vi "Save_EEG_To_XML.vi"(0 "Path to EEG File":path, 1 "SampleRateHz":dbl, 2 "Epoch Duration":dbl, 5 "EEG Refnum in":refnum<data-value>, 7 "ChannelNames in":string[](array[string]), 9 "Trial Info":T1, 11 "error in (no error)":errorcluster) -> (6 "EEG Refnum out":refnum<data-value>, 15 "error out":errorcluster)   [LabVIEW 2016, in "Save Txt To Xml.lvlib"]
uses:
  Save Txt To Xml.lvlib
  Trial_Info.ctl
  _XML_EEG_File_Parser/_vlib/XML_EEG_File.lvclass
  _XML_EEG_File_Parser/_vlib/XML_EEG_Header.ctl
  _XML_EEG_File_Parser/_vlib/XML_EEG_Dataset.ctl
  <vilib>/Waveform/WDTOps.llb/WDT Get Waveform Subset DBL.vi
  <vilib>/measure/madcrms.llb/Basic Averaged DC-RMS for 1 Chan.vi
  _XML_EEG_File_Parser/XML_EEG_File_Parser.lvlib
  <vilib>/measure/NI_MAPro.lvlib
panel:
  # "This VI is a part of BCI Design library, http://www.ru-bci.org \nCopyright © 2020, Sotnikov Peter, All rights reserved. License: GNU GPLv3"
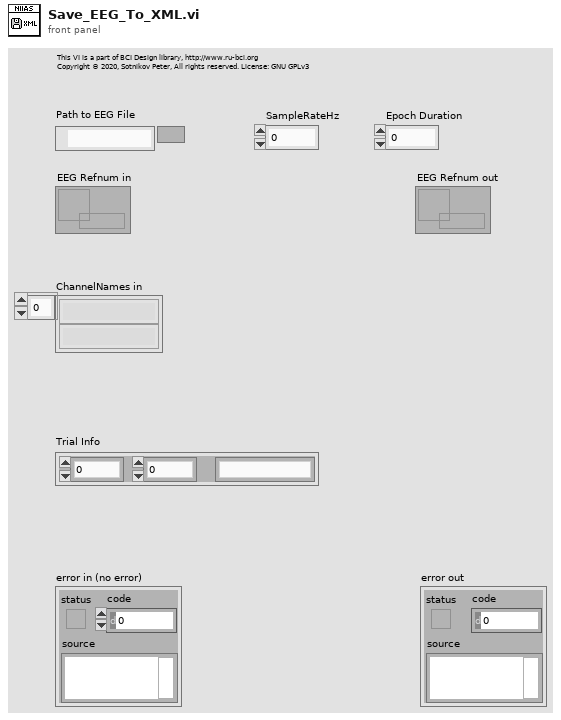
[diagram p1: front panel]
types:
  T1 = typedef "Save Txt To Xml.lvlib/Trial_Info.ctl" = cluster{"Start Position":i32, "End Position":i32, "Class":string}
  T2 = typedef "XML_EEG_File_Parser.lvlib/XML_EEG_Dataset.ctl" = cluster{"Attributes":cluster{"NumberOfSamples":i32, "StartDateTime":timestamp}, "Body":cluster{"MarkerValue":string, "Channels":waveform(dbl)[]}}
  T3 = typedef "XML_EEG_File_Parser.lvlib/XML_EEG_Header.ctl" = cluster{"Attributes":cluster{"ChannelDataType":string, "NumberOfChannels":i32, "SampleRateHz":dbl, "MarkerChannel":i32}, "Body":cluster{"PatientSpecificData":string, "NumberOfDatasets":i32, "Channels":string[]}}
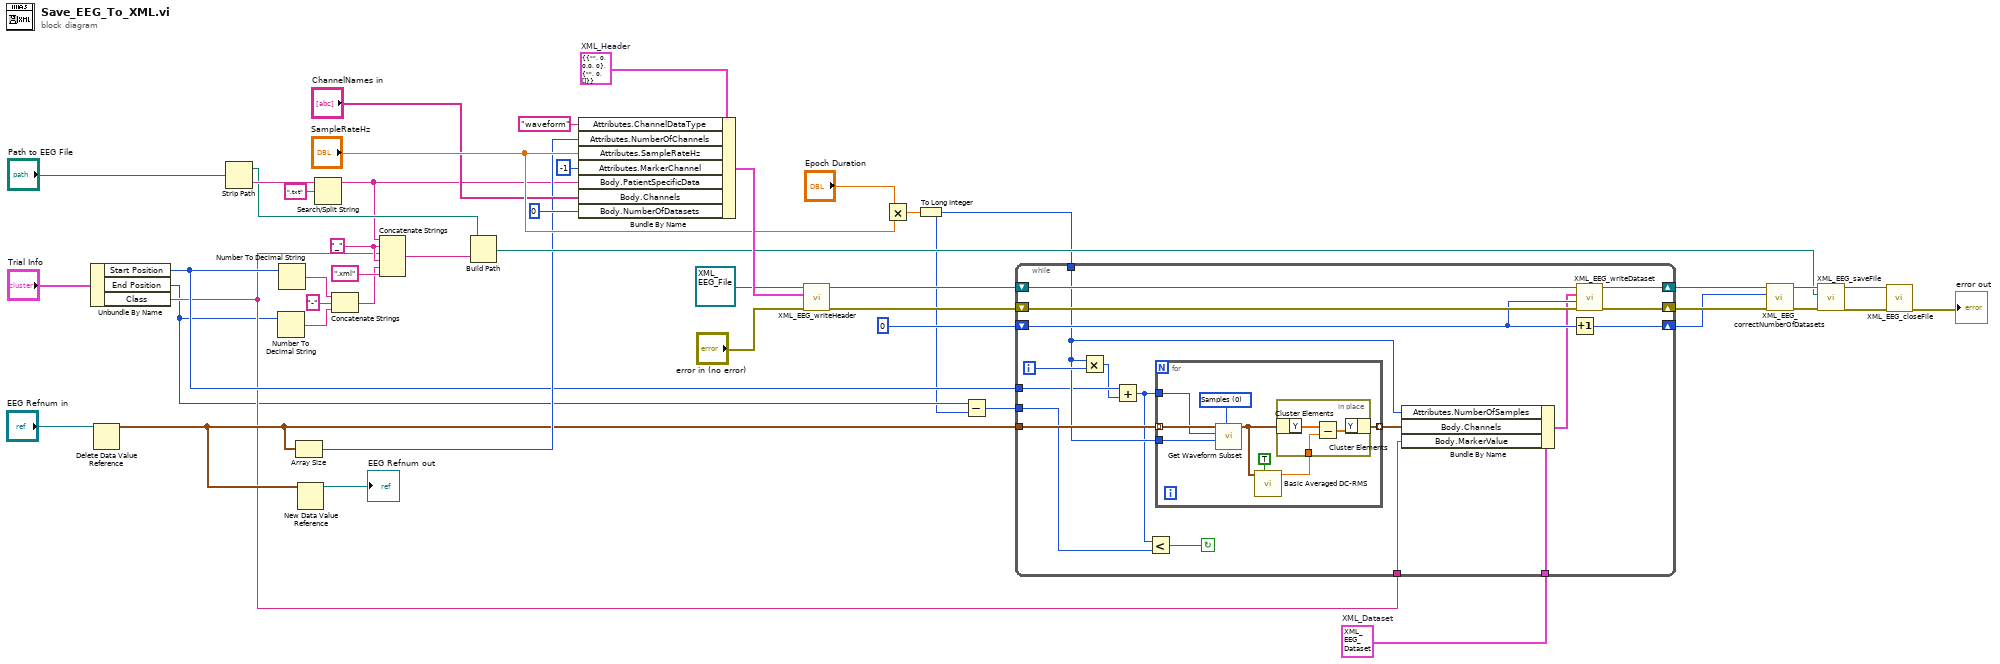
[diagram p0: block diagram]
diagram:
  w9 = "_" ("string")
  w34 = T2 {"Attributes"={"NumberOfSamples"=0, "StartDateTime"=timestamp(0 s since 1904-01-01)}, "Body"={"MarkerValue"="", "Channels"=[]}}  # XML_Dataset
  w46 = T3 {"Attributes"={"ChannelDataType"="", "NumberOfChannels"=0, "SampleRateHz"=0.0, "MarkerChannel"=0}, "Body"={"PatientSpecificData"="", "NumberOfDatasets"=0, "Channels"=[]}}  # XML_Header
  n1 = Unbundle By Name("Trial Info") -> ("Start Position"=w11:i32, "End Position"=w2:i32, "Class"=w4:string)
  n2 = Delete Data Value Reference(data value reference="EEG Refnum in") -> (data value=w15:waveform(dbl)[])  [unwired: 1 in, 1 out]
  n3 = Strip Path(path="Path to EEG File") -> (stripped path=w27:path, name=w42:string)
  n4 = Number To Decimal String(number=w2) -> (decimal integer string=w7:string)  [unwired: 1 in]
  n5 = Number To Decimal String(number=w11) -> (decimal integer string=w8:string)  [unwired: 1 in]
  n6 = Array Size(array=w15) -> (size(s)=w16:i32)
  n7 = New Data Value Reference(data value=w15) -> (data value reference=→"EEG Refnum out":refnum<data-value>)  [unwired: 1 in, 1 out]
  n8 = Search/Split String(string=w42, search string/char (-)=".txt") -> (substring before match=w10:string)  [unwired: 1 in, 2 out]
  n9 = Concatenate Strings(w8, "-" ("string"), w7) -> (w5:string)
  n10 = Concatenate Strings(w10, w9, w4, w9, w5, ".xml" ("string")) -> (w37:string)
  n11 = Build Path(base path=w27, name or relative path=w37) -> (appended path=w28:path)
  n12 = Bundle By Name(cluster=w46, "Attributes.ChannelDataType"="waveform", "Attributes.NumberOfChannels"=w16, "Attributes.SampleRateHz"="SampleRateHz", "Attributes.MarkerChannel"=-1, "Body.PatientSpecificData"=w10, "Body.Channels"="ChannelNames in", "Body.NumberOfDatasets"=0) -> (w45:T3)
  n13 = call "XML_EEG_writeHeader.vi"("error in (no error)"="error in (no error)", "XML_Header"=w45, "XML_EEG_File in"=refnum<class "XML_EEG_File.lvclass"> refnum ("XML_EEG_File_Parser.lvlib:XML_EEG_File.lvclass")) -> ("error out"=w35:errorcluster, "XML_EEG_File out"=w36:refnum<class "XML_EEG_File.lvclass">)  [unwired: 6 in, 1 out]
  n14 = Multiply(x="Epoch Duration", y="SampleRateHz") -> (x*y=w12:dbl)
  n15 = To Long Integer(number=w12) -> (32bit integer=w1:i32)
  n16 = Subtract(x=w2, y=w1) -> (x-y=w3:i32)
  n17 = while {
    tunnel: w34 -> [w62]
    tunnel: w1 -> [w53]
    tunnel: w15 -> [w57]
    shift-right: [w61] -> w32
    shift-left: w36 -> [w64]
    shift-right: [w60] -> w31
    shift-left: w35 -> [w63]
    shift-right: [w59] -> w26
    shift-left: 0 -> [w58]
    tunnel: w11 -> [w52]
    tunnel: w3 -> [w49]
    tunnel: w4 -> [w47]
    i -> [w54]
    stop <- w48 continue-if-true
    n18 = Multiply(x=w53, y=w54) -> (x*y=w51:i32)
    n19 = Add(x=w52, y=w51) -> (x+y=w50:i32)
    n20 = Less?(x=w50, y=w49) -> (x < y?=w48:bool)
    n21 = for {
      tunnel: w57 -> [w72] mode=indexing
      tunnel: w53 -> [w66]
      tunnel: [w67] -> w55 mode=indexing
      tunnel: w50 -> [w65]
      w71 = u16 0 items=["Samples", "Relative Time"] ("start/duration format")
      n22 = call-poly <vilib>:"Get Waveform Subset.vi"("start/duration format"=w71, "duration"=w66, "start samples/time"=w65, "waveform in"=w72) -> ("waveform out"=w69:waveform(dbl))  [unwired: 2 in, 3 out]
      n23 = call-poly <vilib>:"Basic Averaged DC-RMS.vi"("reset"=TRUE, "signal in"=w69) -> ("DC value"=w68:dbl)  [unwired: 6 in, 3 out]
      n24 = in-place {
        in-place-border: w68 -> [w75]
        n25 = in-place-cluster #1(w69) -> ("Y"=w74:dbl[])
        n26 = Subtract(x=w74, y=w75) -> (x-y=w73:dbl[])
        n27 = in-place-cluster #1("Y"=w73) -> (w67:waveform(dbl))
      }
    }
    n28 = Bundle By Name(cluster=w62, "Attributes.NumberOfSamples"=w53, "Body.Channels"=w55, "Body.MarkerValue"=w47) -> (w56:T2)
    n29 = Increment(x=w58) -> (x+1=w59:i32)
    n30 = call "XML_EEG_writeDataset.vi"("error in (no error)"=w63, "DatasetNumber"=w58, "XML_Dataset"=w56, "XML_EEG_File in"=w64) -> ("error out"=w60:errorcluster, "XML_EEG_File out"=w61:refnum<class "XML_EEG_File.lvclass">)  [unwired: 5 in, 1 out]
  }
  n31 = call "XML_EEG_correctNumberOfDatasets.vi"("error in (no error)"=w31, "NumberOfDatasets"=w26, "XML_EEG_File in"=w32) -> ("error out"=w30:errorcluster, "XML_EEG_File out"=w29:refnum<class "XML_EEG_File.lvclass">)  [unwired: 6 in, 1 out]
  n32 = call "XML_EEG_saveFile.vi"("error in (no error)"=w30, "XML file path"=w28, "XML_EEG_File in"=w29) -> ("error out"=w24:errorcluster, "XML_EEG_File out"=w25:refnum<class "XML_EEG_File.lvclass">)  [unwired: 7 in]
  n33 = call "XML_EEG_closeFile.vi"("error in (no error)"=w24, "XML_EEG_File.lvclass"=w25) -> ("error out"=→"error out":errorcluster)  [unwired: 9 in]
